vi "Subvi pixel clock.vi"(9 "Line clock":bool) -> (3 "Pixel clock/Line clock change/FIFO OUT gate":T1, 7 "Pixel clock":bool)   [LabVIEW 2017]
uses:
  <vilib>/rvi/Emulation/niFpgaSctlEmulationGetInTimedLoop.vi
  GV N pixel clock per line.vi
  <vilib>/rvi/Memory/Memory_Emulation/nirvimemoryFastEmulation.vi
  <vilib>/rvi/Memory/Memory_Emulation/nirvimemoryEmulation.vi
  <vilib>/rvi/Emulation/niFpgaEmulationIsFPGAContextNoSignature.vi
  <vilib>/rvi/DataTransferAndStorage/Container/Common/niFpgaContainerGetUniqueNameForEmu.vi
  <vilib>/rvi/Emulation/niFpgaProcessEmulError.vi
  <vilib>/rvi/errors/nirviReportUnexpectedCaseInternalError (U32).vi
  GV FIFO OUT gate.vi
  <vilib>/rvi/DataTransferAndStorage/Container/XNode/niFpgaContainer.xnode
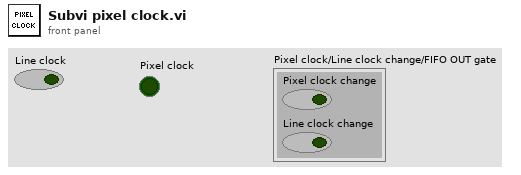
[diagram p1: front panel]
types:
  T1 = cluster{"Pixel clock change":bool, "Line clock change":bool}
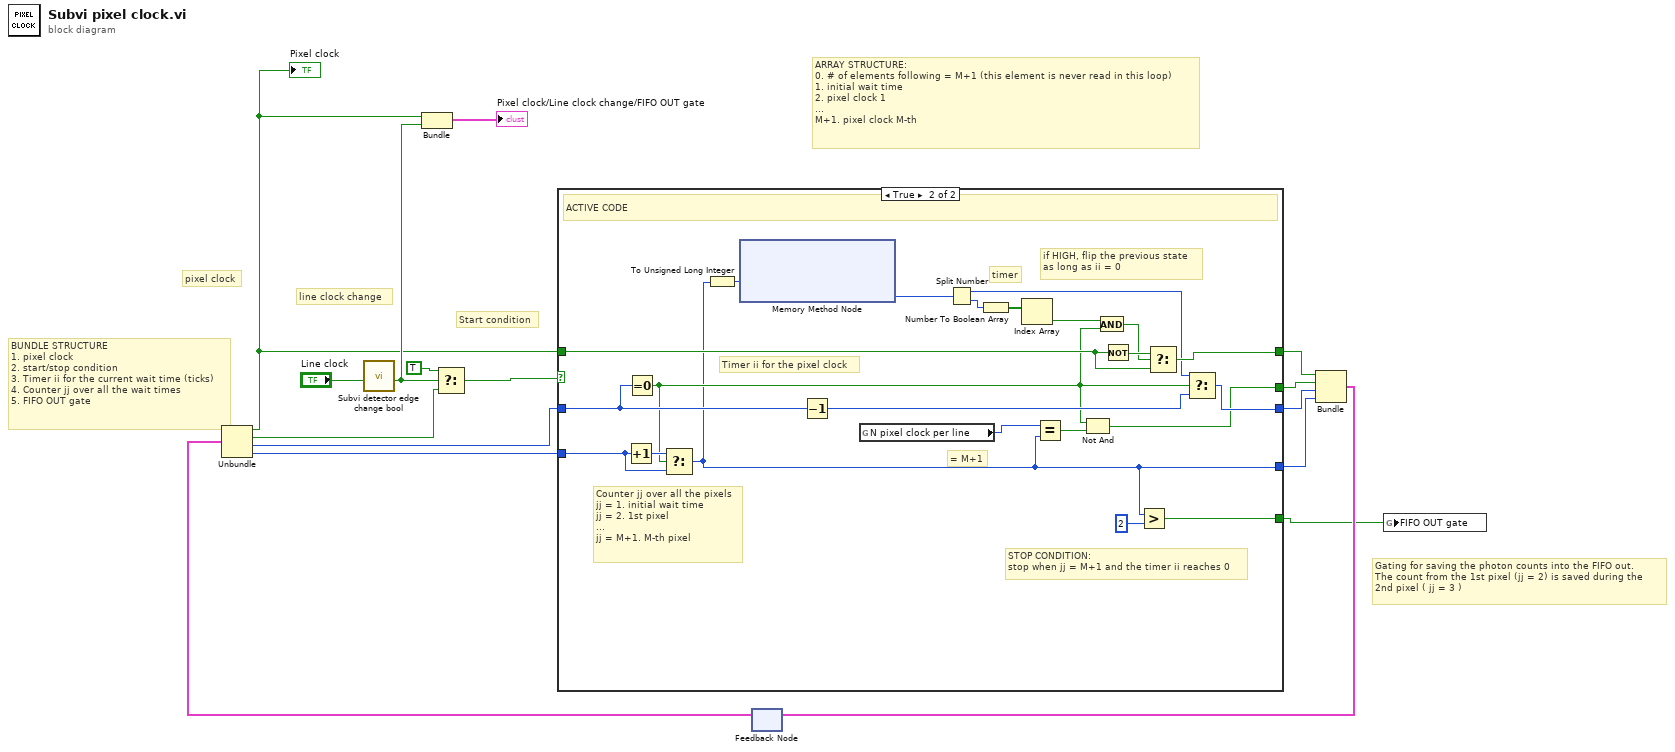
[diagram p0: block diagram]
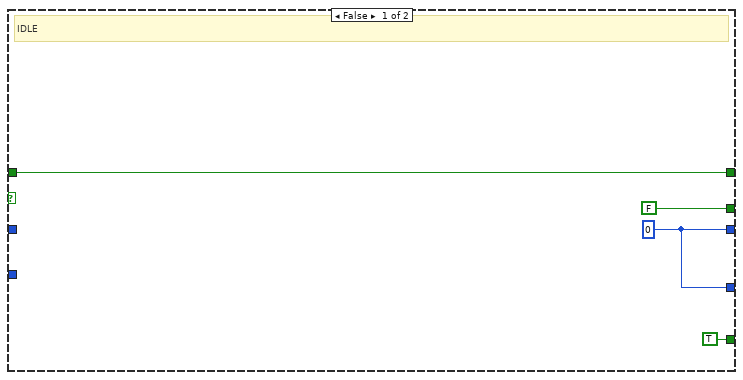
[diagram p2: hidden frame]
diagram:
  # "Gating for saving the photon counts into the FIFO out.\nThe count from the 1st pixel (jj = 2) is saved during the \n2nd pixel ( jj = 3 )"
  # "line clock change"
  # "pixel clock"
  # "BUNDLE STRUCTURE\n1. pixel clock\n2. start/stop condition\n3. Timer ii for the current wait time (ticks)\n4. Counter jj over all the wait times\n5. FIFO OUT gate"
  # "ARRAY STRUCTURE:\n0. # of elements following = M+1 (this element is never read in this loop)\n1. initial wait time \n2. pixel clock 1\n...\nM+1. pixel clock M-th"
  # "Start condition"
  n1 = call "Subvi detector edge change bool.vi"("Input"="Line clock") -> ("Output"=w4:bool)  [unwired: 8 in]
  n2 = feedback #1() -> (w9:cluster{bool, bool, u16, u16})  [unwired: 1 in]
  n3 = Unbundle(w9) -> (w1:bool, w7:bool, w6:u16, w5:u16)
  "Pixel clock" <- w1
  n4 = Bundle(w1, "Output"=w4) -> (→"Pixel clock/Line clock change/FIFO OUT gate":cluster{bool, "Output":bool})  [unwired: 1 in]
  n5 = Select(t=TRUE, s=w4, f=w7) -> (s? t:f=w15:bool)
  n6 = case shown="True" w15 {
    tunnel: [FALSE w25] -> w13
    tunnel: w6 -> [_ w34]
    tunnel: [w20 w37] -> w12
    tunnel: [w18 w38] -> w8
    tunnel: w1 -> [w18 w35]
    tunnel: w5 -> [_ w33]
    tunnel: [w20 w24] -> w11
    tunnel: [TRUE w22] -> w2
    frame False {
      w20 = u16 0
      # "IDLE"
    }
    frame True {
      # "= M+1"
      # "STOP CONDITION:\nstop when jj = M+1 and the timer ii reaches 0"
      # "Counter jj over all the pixels\njj = 1. initial wait time\njj = 2. 1st pixel\n...\njj = M+1. M-th pixel"
      # "timer"
      # "Timer ii for the pixel clock"
      # "if HIGH, flip the previous state\nas long as ii = 0"
      # "ACTIVE CODE"
      n7 = Increment(x=w33) -> (x+1=w42:u16)
      n8 = Equal To 0?(x=w34) -> (x = 0?=w28:bool)
      n9 = Select(t=w42, s=w28, f=w33) -> (s? t:f=w24:u16)
      n10 = To Unsigned Long Integer(number=w24) -> (unsigned 32bit integer=w26:u32)
      n11 = xnode ("Memory Method Node")("Address"=w26) -> ("Data"=w27:u32)  [unwired: 1 in, 1 out]
      n12 = Decrement(x=w34) -> (x-1=w32:u16)
      n13 = global read "GV N pixel clock per line.vi" "N pixel clock per line"() -> (w21:u16)
      n14 = Split Number(x=w27) -> (hi(x)=w36:u16, lo(x)=w40:u16)
      n15 = Number To Boolean Array(number=w40) -> (Boolean array=w41:bool[])
      n16 = Index Array(array=w41) -> (element=w29:bool)  [unwired: 1 in]
      n17 = Equal?(x=w21, y=w24) -> (x = y?=w31:bool)
      n18 = Not And(1:w31, 2:w28) -> (0:w25:bool)
      n19 = And(x=w29, y=w28) -> (x .and. y?=w30:bool)
      n20 = Not(x=w35) -> (.not. x?=w39:bool)
      n21 = Greater?(x=w24, y=u16 2) -> (0:w22:bool)
      n22 = Select(t=w39, s=w30, f=w35) -> (s? t:f=w38:bool)
      n23 = Select(t=w36, s=w28, f=w32) -> (s? t:f=w37:u16)
    }
  }
  n24 = Bundle(w8, w13, w12, w11) -> (w10:cluster{bool, bool, u16, u16})  [unwired: 1 in]
  n25 = feedback-in #1(w10) -> ()
  n26 = global write "GV FIFO OUT gate.vi" "FIFO OUT gate"(w2) -> ()
